vi "Building_Origin_of_Tracks(11)-1.vi"(4 "[IN] Indexes \nfor Jumps":i32[](array[numeric]), 5 "error IN":errorcluster, 6 "[IN] Subtrack":T1, 8 "[IN] Still connected\ntracks in group":T2) -> (0 "error OUT":errorcluster, 1 "[OUT] Subtrack":T1, 2 "[OUT] Last point in subtrack":i32)   [LabVIEW 2013]
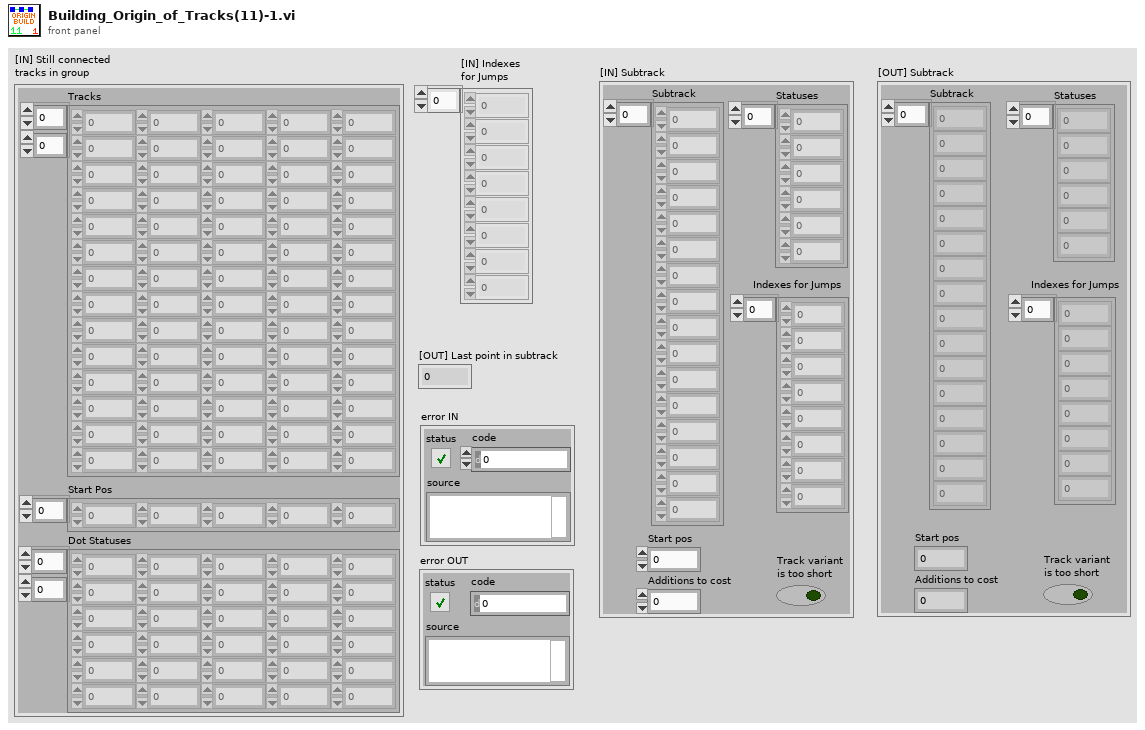
[diagram p1: front panel]
types:
  T1 = cluster{"Subtrack":dbl[], "Statuses":i16[], "Start pos":i32, "Additions to cost":i32, "Track variant \nis too short":bool, "Indexes for Jumps":i32[]}
  T2 = cluster{"Tracks":dbl[][], "Start Pos":i32[], "Dot Statuses":i16[][]}
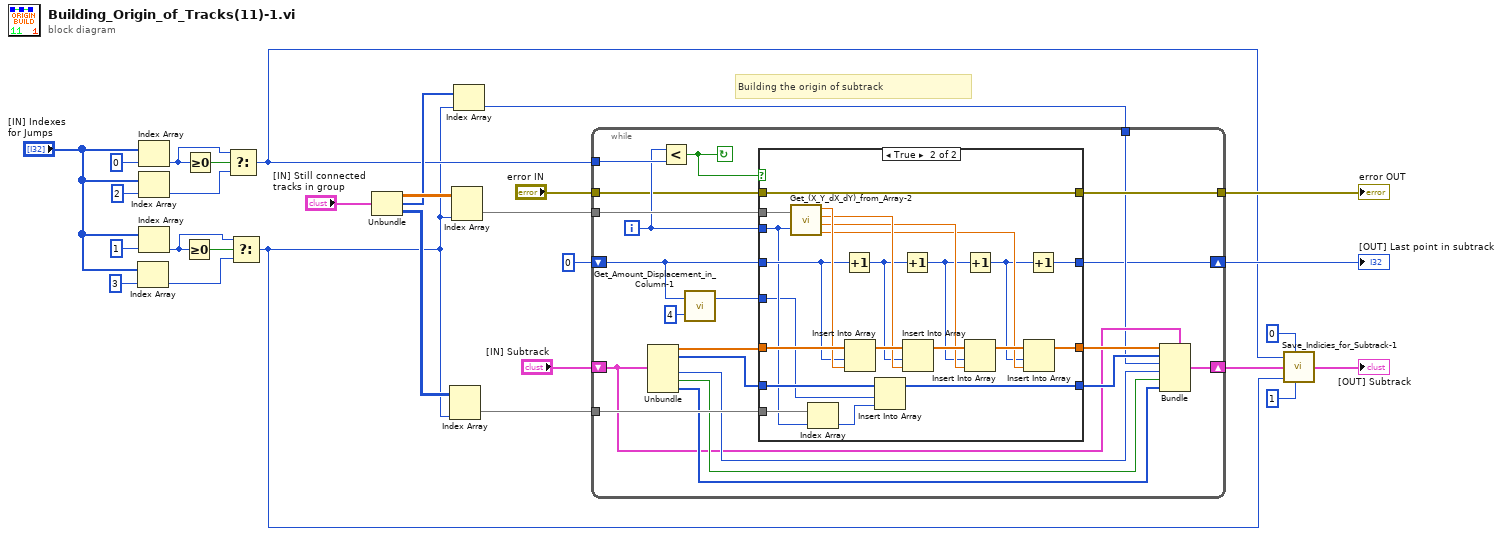
[diagram p0: block diagram]
diagram:
  # "Building the origin of subtrack"
  n1 = Index Array(array="[IN] Indexes \nfor Jumps", index=3) -> (element=w7:i32)
  n2 = Index Array(array="[IN] Indexes \nfor Jumps", index=0) -> (element=w12:i32)
  n3 = Index Array(array="[IN] Indexes \nfor Jumps", index=2) -> (element=w11:i32)
  n4 = Index Array(array="[IN] Indexes \nfor Jumps", index=1) -> (element=w8:i32)
  n5 = Greater Or Equal To 0?(x=w8) -> (x >= 0?=w9:bool)
  n6 = Greater Or Equal To 0?(x=w12) -> (x >= 0?=w13:bool)
  n7 = Select(t=w12, s=w13, f=w11) -> (s? t:f=w4:i32)
  n8 = Select(t=w8, s=w9, f=w7) -> (s? t:f=w1:i32)
  n9 = Unbundle("[IN] Still connected\ntracks in group") -> ("Tracks"=w26:dbl[][], "Start Pos"=w24:i32[], "Dot Statuses"=w22:i16[][])
  n10 = Index Array(array=w22, index (col)=w1) -> (element=w21:i16[])  [unwired: 1 in]
  n11 = Index Array(array=w26, index (col)=w1) -> (element=w25:dbl[])  [unwired: 1 in]
  n12 = Index Array(array=w24, index=w1) -> (element=w23:i32)
  n13 = while {
    tunnel: w25 -> [w50]
    tunnel: w21 -> [w46]
    shift-right: [w41] -> w6
    shift-left: "[IN] Subtrack" -> [w35]
    tunnel: w4 -> [w45]
    tunnel: "error IN" -> [w37]
    tunnel: [w36] -> w19
    tunnel: w23 -> [w34]
    shift-right: [w33] -> w20
    shift-left: 0 -> [w31]
    i -> [w44]
    stop <- w48 continue-if-true
    n14 = Unbundle(w35) -> ("Subtrack"=w49:dbl[], "Statuses"=w47:i16[], "Additions to cost"=w40:i32, "Track variant \nis too short"=w39:bool, "Indexes for Jumps"=w38:i32[])  [unwired: 1 out]
    n15 = Less?(x=w44, y=w45) -> (x < y?=w48:bool)
    n16 = call "Get_Amount_Displacement_in_Column-1.vi"("multiplier"=4, "# Rows"=w31) -> ("Displ amount"=w30:i32)  [unwired: 1 out]
    n17 = case shown="True" w48 {
      tunnel: w50 -> [_ w76]
      tunnel: w49 -> [w53 w75]
      tunnel: w31 -> [w51 w73]
      tunnel: w44 -> [_ w62]
      tunnel: w47 -> [w54 w64]
      tunnel: w46 -> [_ w63]
      tunnel: [w53 w60] -> w43
      tunnel: [w54 w59] -> w42
      tunnel: w37 -> [w52 w58]
      tunnel: [w52 w58] -> w36
      tunnel: [w51 w55] -> w33
      tunnel: w30 -> [_ w57]
      frame False {
      }
      frame True {
        n18 = call "Get_(X_Y_dX_dY)_from_Array-2.vi"("(X,Y,dX,dY)"=w76, "Index of Displacement"=w62) -> ("X"=w74:dbl, "Y"=w71:dbl, "dX"=w68:dbl, "dY"=w65:dbl)
        n19 = Index Array(array=w63, index=w62) -> (element=w61:i16)
        n20 = Increment(x=w73) -> (x+1=w69:i32)
        n21 = Insert Into Array(array=w75, index=w73, new element=w74) -> (w72:dbl[])
        n22 = Insert Into Array(array=w64, index=w57, new element=w61) -> (w59:i16[])
        n23 = Increment(x=w69) -> (x+1=w67:i32)
        n24 = Insert Into Array(array=w72, index=w69, new element=w71) -> (w70:dbl[])
        n25 = Increment(x=w67) -> (x+1=w56:i32)
        n26 = Insert Into Array(array=w70, index=w67, new element=w68) -> (w66:dbl[])
        n27 = Insert Into Array(array=w66, index=w56, new element=w65) -> (w60:dbl[])
        n28 = Increment(x=w56) -> (x+1=w55:i32)
      }
    }
    n29 = Bundle(cluster=w35, "Subtrack"=w43, "Statuses"=w42, "Start pos"=w34, "Additions to cost"=w40, "Track variant \nis too short"=w39, "Indexes for Jumps"=w38) -> (w41:T1)
  }
  "[OUT] Last point in subtrack" <- w20
  "error OUT" <- w19
  n30 = call "Save_Indicies_for_Subtrack-1.vi"("[IN] Index of Origin/Problem \nPoint inside Original Track (X1)"=w4, "[IN] i for X1"=0, "[IN] Subtrack"=w6, "[IN] Index of Track Conta-\nining Origin/Problem (X2)"=w1, "[IN] i for X2"=1) -> ("[OUT] Subtrack"=→"[OUT] Subtrack":T1)
